vi "Make DLL Param(Profile Info).vi"(1 "Profile Info":T1) -> (0 "DLL Parameter":T2)   [LabVIEW 2020, in "KEYENCE LJ-X8000A.lvlib"]
uses:
  KEYENCE LJ-X8000A.lvlib
  Public/Clusters/Profile Info.ctl
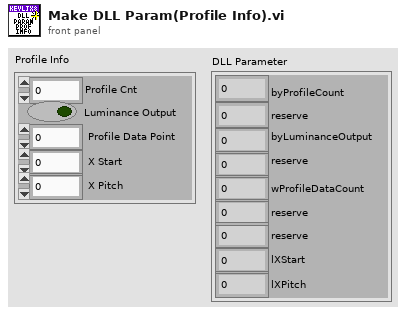
[diagram p1: front panel]
types:
  T1 = typedef "KEYENCE LJ-X8000A.lvlib/Profile Info.ctl" = cluster{"Profile Cnt":u8, "Luminance Output":bool, " Profile Data Point":u16, " X Start":i32, " X Pitch":i32}
  T2 = cluster{"byProfileCount":u8, "reserve":u8, "byLuminanceOutput":u8, "reserve":u8, "wProfileDataCount":u16, "reserve":u8, "reserve":u8, "lXStart":i32, "lXPitch":i32}
  T3 = cluster{"Profile Cnt":u8, "reserve":u8, u8, "reserve":u8, " Profile Data Point":u16, "reserve":u8, "reserve":u8, " X Start":i32, " X Pitch":i32}
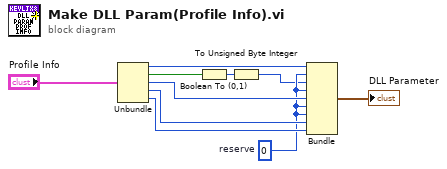
[diagram p0: block diagram]
diagram:
  w2 = u8 0  # reserve
  n1 = Unbundle("Profile Info") -> ("Profile Cnt"=w4:u8, "Luminance Output"=w5:bool, "Profile Data Point"=w7:u16, "X Start"=w8:i32, "X Pitch"=w9:i32)
  n2 = Boolean To (0,1)(Boolean=w5) -> (0, 1=w6:i16)
  n3 = To Unsigned Byte Integer(number=w6) -> (unsigned 8bit integer=w1:u8)
  n4 = Bundle("Profile Cnt"=w4, "reserve"=w2, w1, "reserve"=w2, "Profile Data Point"=w7, "reserve"=w2, "reserve"=w2, "X Start"=w8, "X Pitch"=w9) -> (→"DLL Parameter":T3)  [unwired: 1 in]
